vi "Reverse_Random_Array.vi"() -> ()   [LabVIEW 2020]
panel:
  out "reversed_random_array":dbl[](array[numeric]) format="%#_3g"
  out "random_array":dbl[](array[numeric]) format="%#_3g"
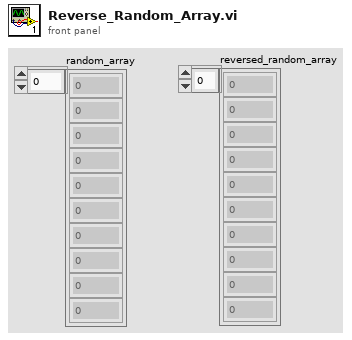
[diagram p1: front panel]
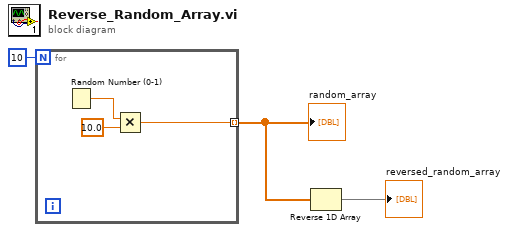
[diagram p0: block diagram]
diagram:
  n1 = for {
    N: 10 -> [_]
    tunnel: [w4] -> w2 mode=indexing
    n2 = Random Number (0-1)() -> (number: 0 to 1=w6:dbl)
    n3 = Multiply(x=w6, y=10.0) -> (x*y=w4:dbl)
  }
  "random_array" <- w2
  n4 = Reverse 1D Array(array=w2) -> (reversed array=→"reversed_random_array":dbl[])
